vi "SetUser.vi"(8 "error in":errorcluster, 10 "User":string, 11 "UserComment in":refnum<class "UserComment.lvclass">) -> (0 "error out":errorcluster, 3 "UserComment out":refnum<class "UserComment.lvclass">)   [LabVIEW 2021, in "ProligentXMLGenerator.lvlib" / "UserComment.lvclass"]
doc: "This value is limited to 255 charactesrs and must no be empty."
uses:
  UserComment.lvclass
  UserComment.lvclass/UserComment.ctl
  Base/NonEmptyString_255/NonEmptyString_255.lvclass
  Base/Attribute/Attribute.lvclass
  C:/Projects/proligent-xml-generator-labview/src/ProligentXMLGenerator/Base/NonEmptyString/NonEmptyString.lvclass
  C:/Projects/proligent-xml-generator-labview/src/ProligentXMLGenerator/Base/String/String.lvclass
  C:/Projects/proligent-xml-generator-labview/src/ProligentXMLGenerator/Base/Attribute/Attribute.lvclass
  C:/Projects/proligent-xml-generator-labview/src/ProligentXMLGenerator/Base/NonEmptyString_255/NonEmptyString_255.lvclass
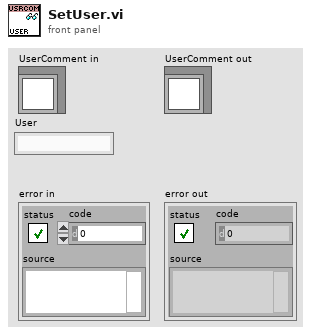
[diagram p1: front panel]
types:
  T1 = typedef "ProligentXMLGenerator.lvlib/UserComment.lvclass/Data.ctl" = cluster{"Name":string, "Comment":refnum<class "NonNullableString_TruncateAt_255.lvclass">, "User":refnum<class "NonEmptyString_255.lvclass">, "Time":refnum<class "DateTime.lvclass">}
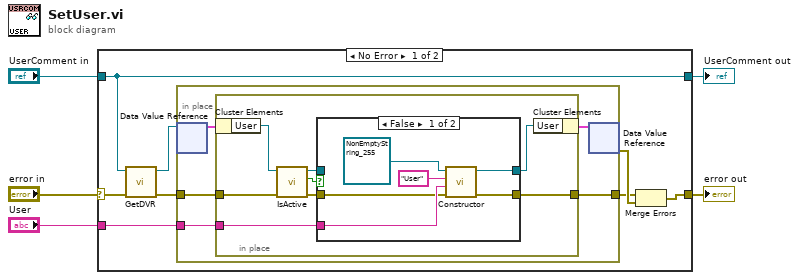
[diagram p0: block diagram]
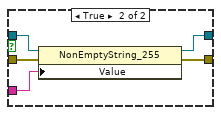
[diagram p2: hidden frame]
diagram:
  n1 = case shown="No Error" "error in" {
    selector: "error in" -> [w11 w38]
    tunnel: "UserComment in" -> [w6 w39]
    tunnel: [w8 w38] -> w3
    tunnel: "User" -> [w7 _]
    tunnel: [w6 w39] -> w1
    frame No Error {
      n2 = call "GetDVR.vi"("error in"=w11, "UserComment"=w6) -> ("error out"=w10:errorcluster, "DVRReference"=w12:refnum<data-value>)  [unwired: 8 in]
      n3 = in-place "In Place Element Structure" {
        in-place-border: w10 -> [w16]
        in-place-border: [w18] -> w9
        in-place-border: w7 -> [w17]
        n4 = in-place-dvr #1(w12) -> (w15:T1)  [unwired: 1 out]
        n5 = in-place "In Place Element Structure" {
          in-place-border: [w26] -> w18
          in-place-border: w17 -> [w25]
          in-place-border: w16 -> [w24]
          n6 = in-place-cluster #2(w15) -> ("User"=w20:refnum<class "NonEmptyString_255.lvclass">)
          n7 = call "IsActive.vi"("error in"=w24, "Attribute in"=w20) -> ("error out"=w21:errorcluster, "IsActive"=w22:bool, "Attribute in"=w23:refnum<class "NonEmptyString_255.lvclass">)  [unwired: 7 in]
          n8 = case shown="False" w22 {
            tunnel: [w28 w37] -> w26
            tunnel: w25 -> [w30 w36]
            tunnel: w23 -> [_ w35]
            tunnel: w21 -> [w29 w34]
            tunnel: [w27 w33] -> w19
            frame False {
              n9 = call-dynamic "Constructor.vi"("error in"=w29, "Value"=w30, "Name"="User", "String in"=refnum<class "NonEmptyString_255.lvclass"> refnum ("User")) -> ("error out"=w28:errorcluster, "String out"=w27:refnum<class "NonEmptyString_255.lvclass">)  [unwired: 6 in]
            }
            frame True {
              n10 = property on="Property Node" class="NonEmptyString_255"(reference=w35, error in=w34, "Value"=w36) -> (reference out=w33:refnum<class "NonEmptyString_255.lvclass">, error out=w37:errorcluster)
            }
          }
          n11 = in-place-cluster #2("User"=w19) -> (w14:T1)
        }
        n12 = in-place-dvr #1(w14) -> (w13:errorcluster)  [unwired: 1 out]
      }
      n13 = Merge Errors(w9, w13) -> (w8:errorcluster)
    }
    frame Error {
    }
  }
  "error out" <- w3
  "UserComment out" <- w1
